vi "ESP Target Test.vi"   [LabVIEW 2014, in "ESP8266 WiFi Wrapper.lvlib"]
uses:
  ESP8266 WiFi Wrapper.lvlib
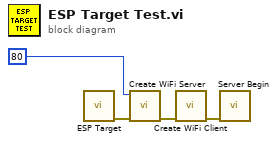
[diagram p0: block diagram]
diagram:
  n1 = call "ESP Target.vi"() -> ("Error Out"=w1:errorcluster)  [unwired: 11 in]
  n2 = call "Create WiFi Server.vi"("Error In"=w1, "Listen Port"=u8 80) -> ("Error Out"=w2:errorcluster)  [unwired: 9 in]
  n3 = call "Create WiFi Client.vi"("Error In"=w2) -> ("Error Out"=w4:errorcluster)  [unwired: 10 in]
  n4 = call "Server Begin.vi"("Error In"=w4) -> ()  [unwired: 10 in, 1 out]
